vi "Test Data Analysis API.vi"() -> ()   [LabVIEW 2016]
doc: "Data Analysis API Tester."
uses:
  Data Analysis.lvlib
  <vilib>/Utility/error.llb/DialogType.ctl
panel:
  in  "REQ Stop Acq":bool
  in  "REQ Signal Selection":bool
  in  "REQ Start Acq":bool
  in  "REQ Wakeup_help_loop":bool
  in  "REQ Initialize Selector":bool
  in  "Show Diagram on Init":bool
  in  "Run as Singleton?":bool
  in  "Show Block Diagram":bool
  in  "Refresh Modules":bool
  out "Active Modules":string[](array[string])
  in  "Stop Module":bool
  in  "Select Module":i32(ring)=-1 caption="Select Module\nTo send Request to" items=["All"=-1]
  in  "Run New Module":bool
  in  "Hide Module Panel":bool
  in  "Show Module Panel":bool
  out "Status":string
  # "This VI tests the API for the Module."
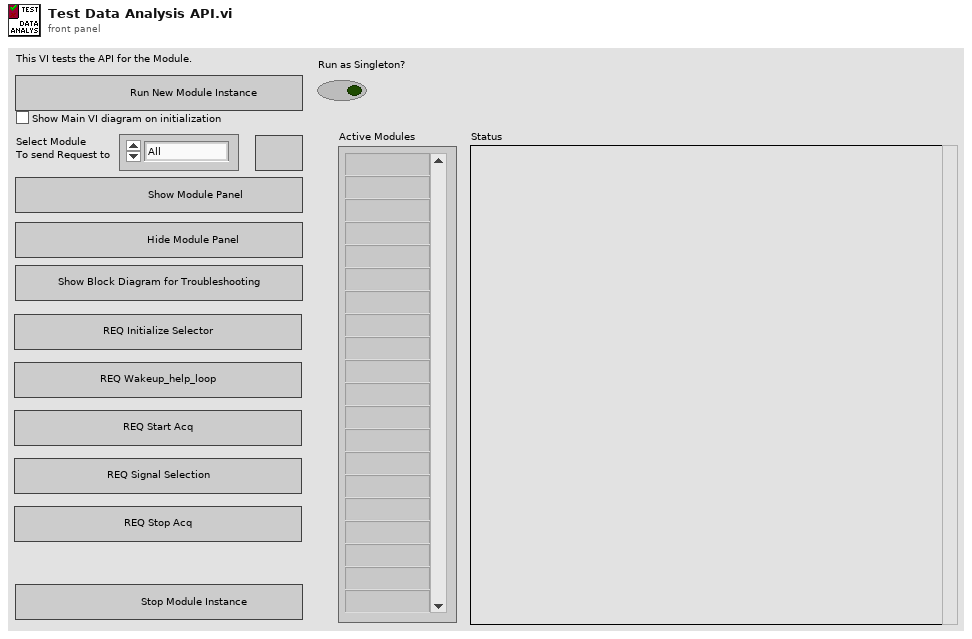
[diagram p1: front panel]
types:
  T1 = typedef "Data Analysis.lvlib/Broadcast Events--cluster.ctl" = cluster{"Module Did Init":refnum<user-event>, "Status Updated":refnum<user-event>, "Error Reported":refnum<user-event>, "Module Did Stop":refnum<user-event>, "Update Module Execution Status":refnum<user-event>}
  T2 = typedef "DialogType.ctl" = u16
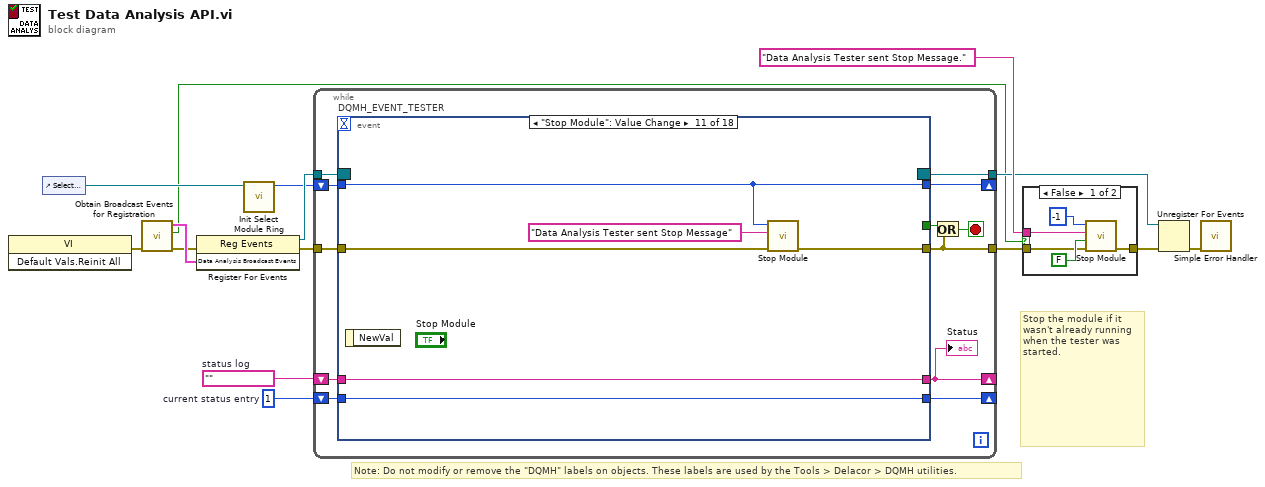
[diagram p0: block diagram]
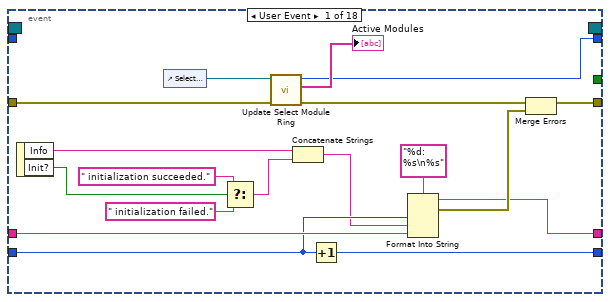
[diagram p3: hidden frame]
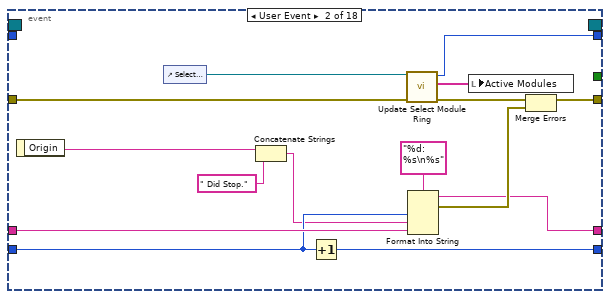
[diagram p4: hidden frame]
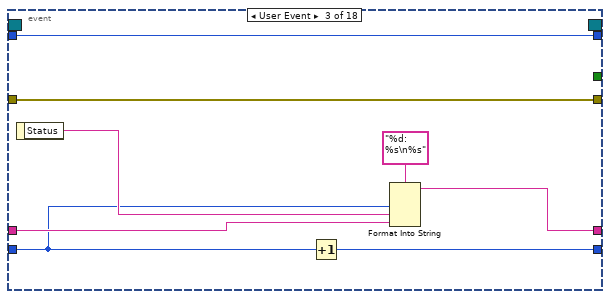
[diagram p5: hidden frame]
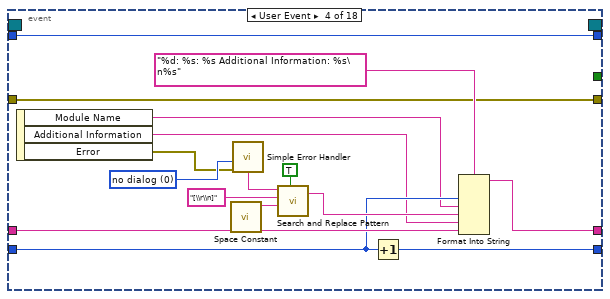
[diagram p6: hidden frame]
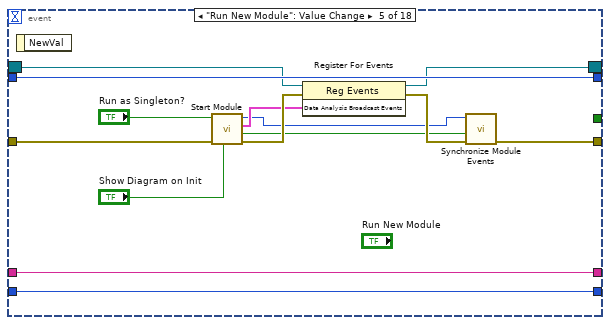
[diagram p7: hidden frame]
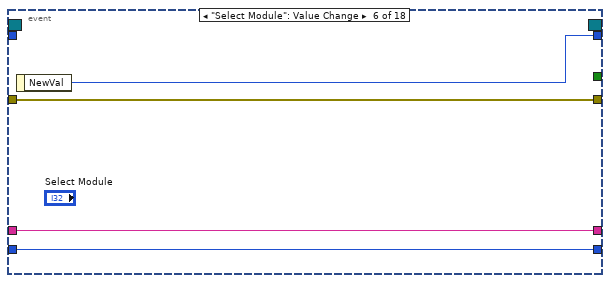
[diagram p8: hidden frame]
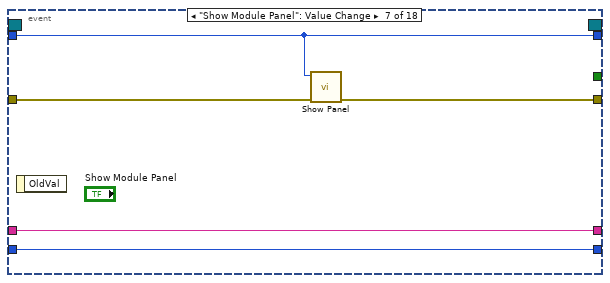
[diagram p9: hidden frame]
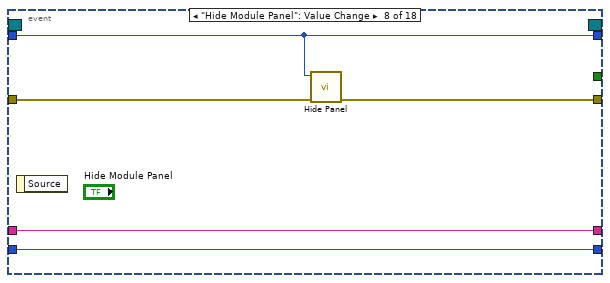
[diagram p10: hidden frame]
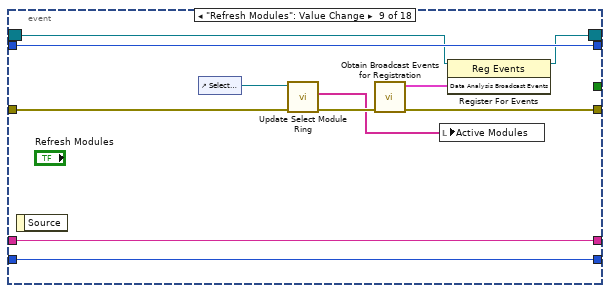
[diagram p11: hidden frame]
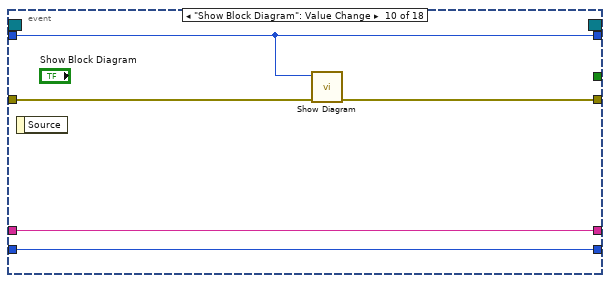
[diagram p12: hidden frame]
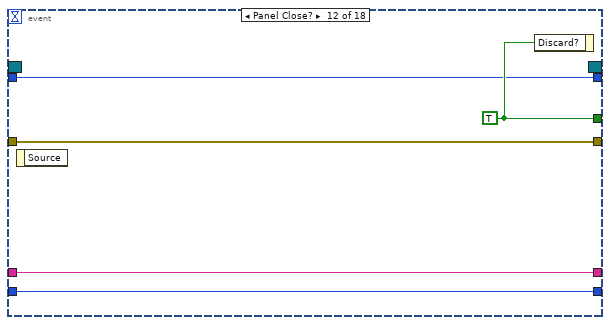
[diagram p13: hidden frame]
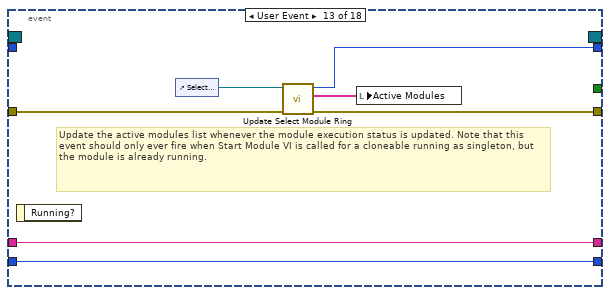
[diagram p14: hidden frame]
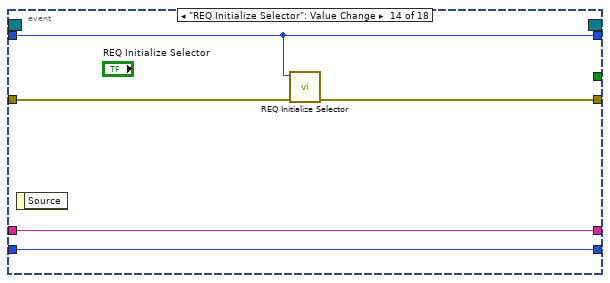
[diagram p15: hidden frame]
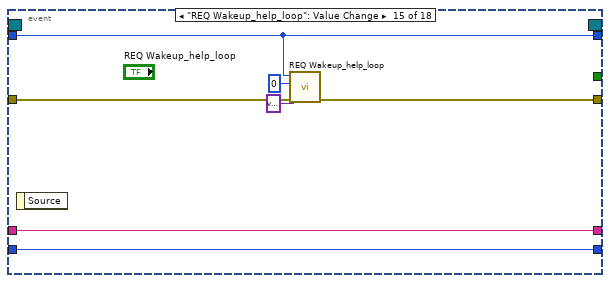
[diagram p16: hidden frame]
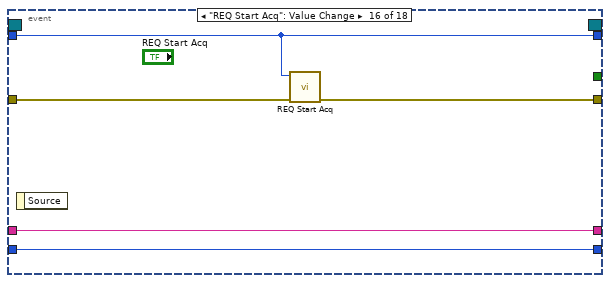
[diagram p17: hidden frame]
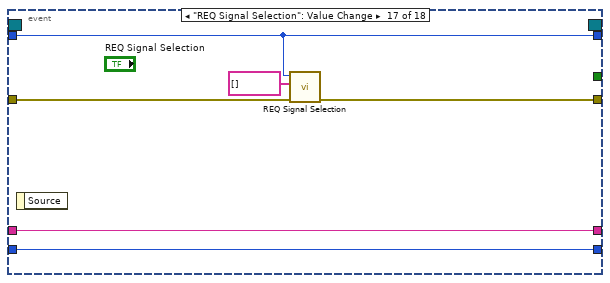
[diagram p18: hidden frame]
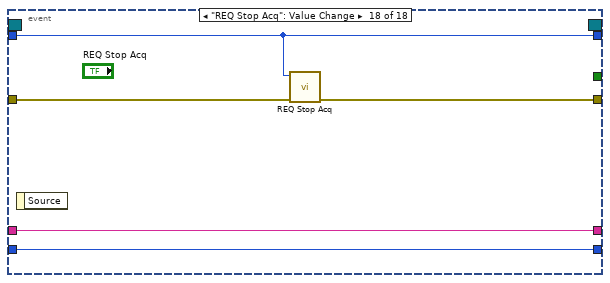
[diagram p19: hidden frame]
diagram:
  w12 = 1  # current status entry
  w13 = ""  # status log
  # "Stop the module if it wasn't already running when the tester was started."
  # "Note: Do not modify or remove the \"DQMH\" labels on objects. These labels are used by the Tools > Delacor > DQMH utilities."
  n1 = invoke class="VI" method="Default Vals.Reinit All"() -> (error out=w5:errorcluster)  [unwired: 3 in, 2 out]
  n2 = control-ref of="Select Module"() -> (w10:refnum<vi>)
  n3 = call "Obtain Broadcast Events for Registration.vi"("error in"=w5) -> ("error out"=w4:errorcluster, "Already running?"=w3:bool, "Data Analysis Broadcast Events"=w9:T1)  [unwired: 8 in]
  n4 = register-events(error in=w4, w9) -> (reference out=w15:refnum<event-registration>, error out=w8:errorcluster)  [unwired: 1 in]
  n5 = call "Init Select Module Ring.vi"("Select Module Ring Ref"=w10) -> ("Value for All Modules"=w11:i32)  [unwired: 8 in, 2 out]
  n6 = while {
    tunnel: w15 -> [w27]
    tunnel: [w16] -> w2
    tunnel: w8 -> [w25]
    shift-right: [w21] -> _
    shift-left: w13 -> [w23]
    shift-right: [w22] -> _
    shift-left: w12 -> [w24]
    shift-right: [w18] -> _
    shift-left: w11 -> [w19]
    tunnel: [w17] -> w6
    stop <- w20 stop-if-true
    n7 = event "DQMH_EVENT_TESTER" shown="[10] \"Stop Module\": Value Change" {
      selector: w27 -> [_ _ _ _ w92 _ _ _ w118 _ _ _ _ _ _ _ _ _]
      dyn-events: [_ _ _ _ w91 _ _ _ w117 _ _ _ _ _ _ _ _ _] -> w17
      timeout: _ -> [_ _ _ _ _ _ _ _ _ _ _ _ _ _ _ _ _ _]
      tunnel: [_ _ _ _ _ _ _ _ _ _ _ w139 _ _ _ _ _ _] -> w26
      tunnel: [w35 w52 w68 w72 w90 w102 w106 w111 w114 w125 w130 w138 w142 w148 w155 w160 w166 w171] -> w16
      tunnel: w25 -> [w37 w54 w68 w72 w93 w102 w107 w112 w119 w128 w131 w138 w143 w151 w158 w163 w169 w174]
      tunnel: w24 -> [w42 w57 w61 w75 w95 w100 w104 w109 w122 w126 w133 w136 w145 w149 w156 w161 w167 w172]
      tunnel: w23 -> [w43 w58 w64 w76 w96 w101 w105 w110 w123 w127 w134 w137 w146 w150 w157 w162 w168 w173]
      tunnel: [w40 w55 w65 w74 w96 w101 w105 w110 w123 w127 w134 w137 w146 w150 w157 w162 w168 w173] -> w21
      tunnel: [w41 w56 w67 w73 w95 w100 w104 w109 w122 w126 w133 w136 w145 w149 w156 w161 w167 w172] -> w22
      tunnel: w19 -> [_ _ w62 w84 w94 _ w103 w108 w121 w124 w132 w135 _ w147 w154 w159 w165 w170]
      tunnel: [w32 w49 w62 w84 w94 w99 w103 w108 w121 w124 w132 w135 w141 w147 w154 w159 w165 w170] -> w18
      event User Event {
        n8 = event-data() -> ("Info"=w39:string, "Init?"=w29:bool)  [unwired: 1 in]
        n9 = control-ref of="Select Module"() -> (w34:refnum<vi>)
        n10 = Select(t=" initialization succeeded.", s=w29, f=" initialization failed.") -> (s? t:f=w28:string)
        n11 = call "Update Select Module Ring.vi"("error in (no error)"=w37, "Select Module Ring Ref"=w34) -> ("error out"=w36:errorcluster, "Active Modules (Array)"=→"Active Modules":string[], "New Module Ring Value"=w32:i32)  [unwired: 7 in]
        n12 = Concatenate Strings(w39, w28) -> (w38:string)
        n13 = Increment(x=w42) -> (x+1=w41:i32)
        n14 = Format Into String(format string="%d: %s\n%s", w42, w38, w43) -> (resulting string=w40:string, error out=w45:errorcluster)  [unwired: 2 in]
        n15 = Merge Errors(w36, w45) -> (w35:errorcluster)
      }
      event User Event {
        n16 = event-data() -> ("Origin"=w47:string)  [unwired: 1 in]
        n17 = control-ref of="Select Module"() -> (w51:refnum<vi>)
        n18 = Concatenate Strings(w47, " Did Stop.") -> (w46:string)
        n19 = Increment(x=w57) -> (x+1=w56:i32)
        n20 = call "Update Select Module Ring.vi"("error in (no error)"=w54, "Select Module Ring Ref"=w51) -> ("error out"=w53:errorcluster, "Active Modules (Array)"=w50:string[], "New Module Ring Value"=w49:i32)  [unwired: 7 in]
        n21 = Format Into String(format string="%d: %s\n%s", w57, w46, w58) -> (resulting string=w55:string, error out=w60:errorcluster)  [unwired: 2 in]
        n22 = local write "Active Modules"(w50) -> ()
        n23 = Merge Errors(w53, w60) -> (w52:errorcluster)
      }
      event User Event {
        n24 = event-data() -> ("Status"=w63:string)  [unwired: 1 in]
        n25 = Increment(x=w61) -> (x+1=w67:i32)
        n26 = Format Into String(format string="%d: %s\n%s", w61, w63, w64) -> (resulting string=w65:string)  [unwired: 2 in, 1 out]
      }
      event User Event {
        w77 = T2 0 items=["no dialog", "OK message", "continue or stop message", "OK message + warnings", "continue/stop + warnings"] ("type of dialog (OK msg:1)")
        n27 = event-data() -> ("Module Name"=w71:string, "Additional Information"=w70:string, "Error"=w69:errorcluster)  [unwired: 1 in]
        n28 = call <vilib>:"Space Constant.vi"() -> ("String"=w81:string)
        n29 = call <vilib>:"Simple Error Handler.vi"("type of dialog (OK msg:1)"=w77, "error in (no error)"=w69) -> ("message"=w78:string)  [unwired: 3 in, 4 out]
        n30 = call <vilib>:"Search and Replace Pattern.vi"("string"=w78, "regular expression (\"\")"="[\\r\\n]" ("regular expression (\"\")"), "replace string (\"\")"=w81, "replace all? (F)"=TRUE ("replace all CR/LF with spaces")) -> ("result string"=w79:string)  [unwired: 1 in, 1 out]
        n31 = Increment(x=w75) -> (x+1=w73:i32)
        n32 = Format Into String(format string="%d: %s: %s Additional Information: %s\n%s", w75, w71, w79, w70, w76) -> (resulting string=w74:string)  [unwired: 2 in, 1 out]
      }
      event "Run New Module": Value Change {
        n33 = event-data() -> ()  [unwired: 1 in, 1 out]
        n34 = call "Start Module.vi"("Show Main VI Diagram on Init (F)"="Show Diagram on Init", "error in"=w93, "Run as Singleton? (F)"="Run as Singleton?") -> ("error out"=w97:errorcluster, "Wait for Event Sync?"=w89:bool, "Data Analysis Broadcast Events"=w88:T1, "Module ID"=w85:i32)  [unwired: 5 in]
        n35 = register-events(reference=w92, error in=w97, w88) -> (reference out=w91:refnum<event-registration>, error out=w98:errorcluster)
        n36 = call "Synchronize Module Events.vi"("error in"=w98, "Wait for Event Sync?"=w89, "Module ID in"=w85) -> ("error out"=w90:errorcluster)  [unwired: 7 in, 1 out]
      }
      event "Select Module": Value Change {
        n37 = event-data() -> ("NewVal"=w99:i32)  [unwired: 1 in]
      }
      event "Show Module Panel": Value Change {
        n38 = event-data() -> ()  [unwired: 1 in, 1 out]
        n39 = call "Show Panel.vi"("error in (no error)"=w107, "Module ID"=w103) -> ("error out"=w106:errorcluster)  [unwired: 9 in]
      }
      event "Hide Module Panel": Value Change {
        n40 = event-data() -> ()  [unwired: 1 in, 1 out]
        n41 = call "Hide Panel.vi"("error in (no error)"=w112, "Module ID"=w108) -> ("error out"=w111:errorcluster)  [unwired: 9 in]
      }
      event "Refresh Modules": Value Change {
        n42 = event-data() -> ()  [unwired: 1 in, 1 out]
        n43 = control-ref of="Select Module"() -> (w120:refnum<vi>)
        n44 = call "Update Select Module Ring.vi"("error in (no error)"=w119, "Select Module Ring Ref"=w120) -> ("error out"=w115:errorcluster, "Active Modules (Array)"=w113:string[])  [unwired: 7 in, 1 out]
        n45 = call "Obtain Broadcast Events for Registration.vi"("error in"=w115) -> ("error out"=w114:errorcluster, "Data Analysis Broadcast Events"=w116:T1)  [unwired: 8 in, 1 out]
        n46 = local write "Active Modules"(w113) -> ()
        n47 = register-events(reference=w118, w116) -> (reference out=w117:refnum<event-registration>)  [unwired: 1 in, 1 out]
      }
      event "Show Block Diagram": Value Change {
        n48 = event-data() -> ()  [unwired: 1 in, 1 out]
        n49 = call "Show Diagram.vi"("error in (no error)"=w128, "Module ID"=w124) -> ("error out"=w125:errorcluster)  [unwired: 9 in]
      }
      event "Stop Module": Value Change {
        n50 = event-data() -> ()  [unwired: 1 in, 1 out]
        n51 = call "Stop Module.vi"("error in"=w131, "Origin"="Data Analysis Tester sent Stop Message", "Module ID"=w132) -> ("error out"=w130:errorcluster)  [unwired: 8 in]
      }
      event Panel Close? {
        w139 = TRUE ("Discard?")
        n52 = event-data() -> ()  [unwired: 1 in, 1 out]
        n53 = event-data("Discard?"=w139) -> ()  [unwired: 1 in, 1 out]
      }
      event User Event {
        # "Update the active modules list whenever the module execution status is updated. Note that this event should only ever fire when Start Module VI is called for a cloneable running as singleton, but the module is already running."
        n54 = event-data() -> ()  [unwired: 1 in, 1 out]
        n55 = control-ref of="Select Module"() -> (w144:refnum<vi>)
        n56 = call "Update Select Module Ring.vi"("error in (no error)"=w143, "Select Module Ring Ref"=w144) -> ("error out"=w142:errorcluster, "Active Modules (Array)"=w140:string[], "New Module Ring Value"=w141:i32)  [unwired: 7 in]
        n57 = local write "Active Modules"(w140) -> ()
      }
      event "REQ Initialize Selector": Value Change {
        n58 = event-data() -> ()  [unwired: 1 in, 1 out]
        n59 = call "REQ Initialize Selector.vi"("error in"=w151, "Module ID"=w147) -> ("error out"=w148:errorcluster)  [unwired: 9 in]
      }
      event "REQ Wakeup_help_loop": Value Change {
        n60 = event-data() -> ()  [unwired: 1 in, 1 out]
        n61 = call "REQ Wakeup_help_loop.vi"("error in"=w158, "Message Data"=variant, "Timeout"=0, "Module ID"=w154) -> ("error out"=w155:errorcluster)  [unwired: 7 in]
      }
      event "REQ Start Acq": Value Change {
        n62 = event-data() -> ()  [unwired: 1 in, 1 out]
        n63 = call "REQ Start Acq.vi"("error in"=w163, "Module ID"=w159) -> ("error out"=w160:errorcluster)  [unwired: 9 in]
      }
      event "REQ Signal Selection": Value Change {
        n64 = event-data() -> ()  [unwired: 1 in, 1 out]
        n65 = call "REQ Signal Selection.vi"("error in"=w169, "Signal Selection"=string[] [], "Module ID"=w165) -> ("error out"=w166:errorcluster)  [unwired: 8 in]
      }
      event "REQ Stop Acq": Value Change {
        n66 = event-data() -> ()  [unwired: 1 in, 1 out]
        n67 = call "REQ Stop Acq.vi"("error in"=w174, "Module ID"=w170) -> ("error out"=w171:errorcluster)  [unwired: 9 in]
      }
    }
    "Status" <- w21
    n68 = Or(x=w26, y=w16) -> (x .or. y?=w20:bool)
  }
  n69 = case shown="False" w3 {
    tunnel: [w179 w180] -> w14
    tunnel: "Data Analysis Tester sent Stop Message." ("Origin") -> [w178 _]
    tunnel: w2 -> [w175 w180]
    frame False {
      n70 = call "Stop Module.vi"("error in"=w175, "Wait for Module to stop? (F)"=FALSE ("Wait for Module to stop?"), "Origin"=w178, "Module ID"=-1 ("Stop all")) -> ("error out"=w179:errorcluster)  [unwired: 7 in]
    }
    frame True {
    }
  }
  n71 = Unregister For Events(event registration refnum=w6, error in=w14) -> (error out=w1:errorcluster)
  n72 = call <vilib>:"Simple Error Handler.vi"("error in (no error)"=w1) -> ()  [unwired: 4 in, 5 out]
